vi "niScope Configure Trigger Output.vi"(0 "instrument handle":refnum<k15>, 1 "trigger event":T2 items=["None", "Stop Trigger", "Start Trigger", "End of Acquisition", "End of Record"], 5 "trigger output source":T1 items=["None"=0, "RTSI 0"=1, "RTSI 1"=2, "RTSI 2"=3, "RTSI 3"=4, "RTSI 4"=5, "RTSI 5"=6, "RTSI 6"=7, "RTSI 7"=18, "PFI 0"=19, "PFI 1"=8, "PFI 2"=9, "PXI Star Trigger"=17], 11 "error in":errorcluster) -> (4 "instrument handle out":refnum<k15>, 15 "error out":errorcluster)   [LabVIEW 2013]
doc: "Configures the digitizer to generate a signal pulse that other digitizers can detect when configured for digital triggering.\n\n<B>NOTE:</B> For Traditional NI-DAQ devices, exported signals are still present in the route after the session is closed. You must clear the route before closing the session, or call\n\nFor NI-DAQmx devices, closing the session clears the routes. However, if you want to clear the routes before closing the session, call this VI again, routing the Stop Trigger to None.\n\nThis VI is obsolete. Consider using niScope Export Signal instead."
uses:
  <instrlib>/niScope/Controls/niScope trigger event.ctl
  <instrlib>/niScope/Controls/niScope trigger output source.ctl
  niScope_32.dll
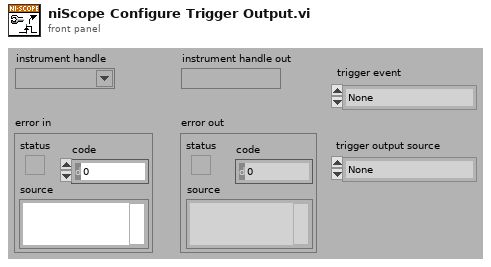
[diagram p1: front panel]
types:
  T1 = typedef "niScope trigger output source.ctl" = u16
  T2 = typedef "niScope trigger event.ctl" = u16
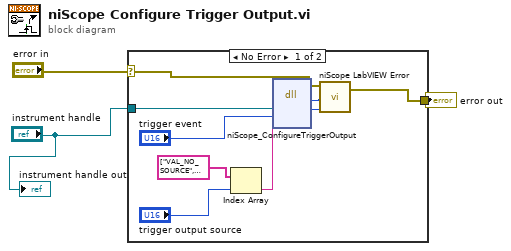
[diagram p0: block diagram]
diagram:
  n1 = case shown="No Error" "error in" {
    selector: "error in" -> [w4 w13]
    tunnel: [w5 w13] -> w3
    tunnel: "instrument handle" -> [w12 _]
    frame No Error {
      n2 = Index Array(array=string[] ["VAL_NO_SOURCE", "VAL_RTSI_0", "VAL_RTSI_1", "VAL_RTSI_2", "VAL_RTSI_3", "VAL_RTSI_4", "VAL_RTSI_5", "VAL_RTSI_6", "VAL_PFI_1", "VAL_PFI_2", "VAL_TTL0", "VAL_TTL1", "VAL_TTL2", "VAL_TTL3", "VAL_TTL4", "VAL_TTL5", "VAL_TTL6", "VAL_PXI_STAR", "VAL_RTSI_7", "VAL_PFI_0"] ("trigger source array"), index="trigger output source") -> (element=w8:string)
      n3 = dll-call lib="niScope_*.*" fn="niScope_ConfigureTriggerOutput"("instrument handle"=w12, "triggerEvent"="trigger event", "triggerOutput"=w8) -> ("status"=w6:i32, "instrument handle"=w7:u32)  [unwired: 5 in, 2 out]
      n4 = call <instrlib>:"niScope LabVIEW Error.vi"("instrument handle"=w7, "niScope error code (0)"=w6, "error in (no error)"=w4) -> ("error out"=w5:errorcluster)  [unwired: 2 in]
    }
    frame Error {
    }
  }
  "error out" <- w3
  "instrument handle out" <- "instrument handle"
